vi "FGV T90.vi"(6 "Aktion":T1, 8 "error in (no error)":errorcluster caption="Fehler (Eingang, kein Fehler)", 9 "Entnahme aktiv":u16, 10 "N2 Spülen aktiv":u16, 11 "T90 aktiv":u16) -> (0 "error out":errorcluster caption="Fehler (Ausgang)", 1 "Entnahme aktiv":bool, 2 "N2 Spülen aktiv":bool, 3 "T90 aktiv":bool)   [LabVIEW 2020, in "Allgemein.lvlib"]
uses:
  Allgemein.lvlib
  Aktion FGV T90.ctl
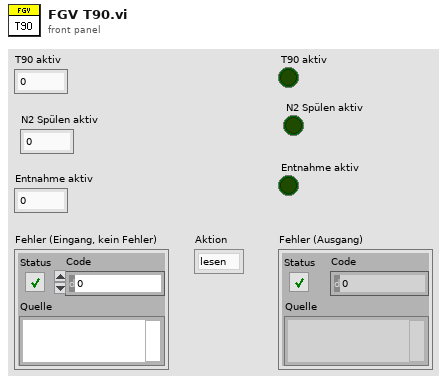
[diagram p1: front panel]
types:
  T1 = typedef "Allgemein.lvlib/Aktion FGV T90.ctl" = enum16{"lesen", "schreiben"}
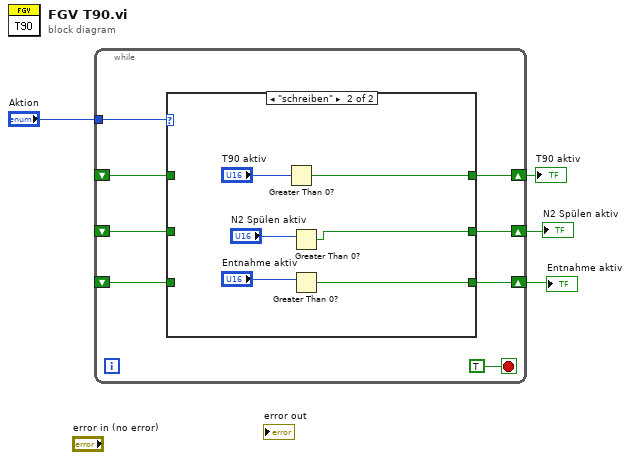
[diagram p0: block diagram]
diagram:
  n1 = while {
    tunnel: "Aktion" -> [w11]
    shift-right: [w10] -> w3
    shift-left: _ -> [w9]
    shift-right: [w8] -> w1
    shift-left: _ -> [w7]
    shift-right: [w6] -> w2
    shift-left: _ -> [w5]
    stop <- TRUE stop-if-true
    n2 = case shown="\"schreiben\"" w11 {
      tunnel: [w15 w20] -> w10
      tunnel: w9 -> [w15 _]
      tunnel: [w14 w16] -> w8
      tunnel: w7 -> [w14 _]
      tunnel: [w13 w18] -> w6
      tunnel: w5 -> [w13 _]
      frame "lesen", Default {
      }
      frame "schreiben" {
        n3 = Greater Than 0?(x="T90 aktiv") -> (x > 0?=w20:bool)
        n4 = Greater Than 0?(x="N2 Spülen aktiv") -> (x > 0?=w16:bool)
        n5 = Greater Than 0?(x="Entnahme aktiv") -> (x > 0?=w18:bool)
      }
    }
  }
  "T90 aktiv" <- w3
  "Entnahme aktiv" <- w2
  "N2 Spülen aktiv" <- w1
